vi "Create Icon Layer New.vi"(8 "error in (no error)":errorcluster, 9 "Template data":T5 {"Opacity" scale=0.0..100.0}, 10 "Icon data":T1={"Text Visible?"=FALSE, "Text Opacity"=0, "Templ Visible?"=FALSE, "Templ Opacity"=0, "Relative Path from 1 to 2"=path "", "Image"=bytes[0], "All User Layers"=[], "Body Text"={"Line 1 text"="", "Line 2 text"="", "Line 3 text"="", "Line 4 text"="", "Line 1 color"=0, "Line 2 color"=0, "Line 3 color"=0, "Line 4 color"=0, "Body Text Spec"={"Font"="", "Alignment"=0, "Size"=3}, "Center text vertically"=FALSE, "Capitalize Text"=FALSE}} {"Body Text"."Body Text Spec"."Alignment" items=["left", "center", "right"]}, 11 "Text data":T5 {"Opacity" scale=0.0..100.0}) -> (0 "error out":errorcluster, 3 "Icon out":refnum<class "Icon.lvclass">)   [LabVIEW 2020, in "VI Properties Editor.lvlib"]
doc: "Create an Icon Layer with the given data from the LabVIEW Icon Data."
uses:
  VI Properties Editor.lvlib
  <vilib>/LabVIEW Icon API/lv_icon/Classes/Icon/Icon.lvclass
  <vilib>/LabVIEW Icon API/lv_icon/Classes/Layer/Layer.lvclass
  <vilib>/LabVIEW Icon API/lv_icon/Classes/Icon Framework/Icon Framework.lvclass
  <vilib>/LabVIEW Icon API/lv_icon/Controls/LayerType.ctl
  <vilib>/LabVIEW Icon API/lv_icon/Controls/Graphic.ctl
  <vilib>/LabVIEW Icon API/lv_icon/lv_icon.lvlib
  <vilib>/LabVIEW Icon API/lv_icon/Controls/Pathes.ctl
  <vilib>/LabVIEW Icon API/lv_icon/Controls/Layer.ctl
  <vilib>/LabVIEW Icon API/lv_icon/Controls/Font.ctl
  <vilib>/LabVIEW Icon API/lv_icon/Controls/Alignment.ctl
  <vilib>/LabVIEW Icon API/lv_icon/Controls/BodyText.ctl
  <vilib>/LabVIEW Icon API/lv_icon/Controls/LabVIEW Icon Stored Information.ctl
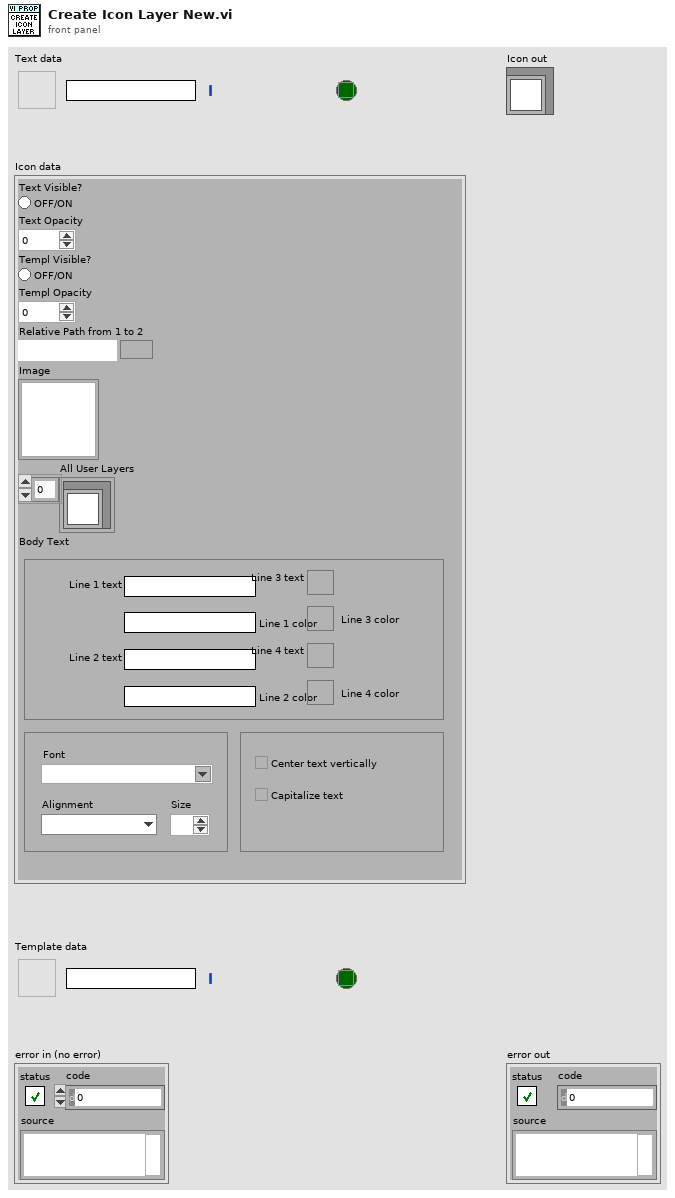
[diagram p1: front panel]
types:
  T1 = typedef "LabVIEW Icon Stored Information.ctl" = cluster{"Text Visible?":bool, "Text Opacity":u8, "Templ Visible?":bool, "Templ Opacity":u8, "Relative Path from 1 to 2":path, "Image":picture, "All User Layers":refnum<class "Layer.lvclass">[], "Body Text":T2}
  T2 = typedef "BodyText.ctl" = cluster{"Line 1 text":string, "Line 2 text":string, "Line 3 text":string, "Line 4 text":string, "Line 1 color":u32, "Line 2 color":u32, "Line 3 color":u32, "Line 4 color":u32, "Body Text Spec":cluster{"Font":T3, "Alignment":T4, "Size":u8}, "Center text vertically":bool, "Capitalize Text":bool}
  T3 = typedef "Font.ctl" = string
  T4 = typedef "Alignment.ctl" = u16
  T5 = typedef "Layer.ctl" = cluster{"LayerIcon":picture, "LayerName":string, "Opacity":u8, "Visibility?":bool}
  T6 = typedef "Pathes.ctl" = enum16{"Root Path", "Icon Templates", "Icon Templates VI", "Icon Templates Lib", "Glyphs"}
  T7 = typedef "Graphic.ctl" = cluster{"Rectangle":cluster{"left":i16, "top":i16, "right":i16, "bottom":i16}, "Path":path, "Image":picture, "Filter":string, "FileName":string}
  T8 = typedef "LayerType.ctl" = enum16{"Graphic", "Text", "Tool", "Graphic Drop"}
  T9 = typedef "imagedata.ctl" = cluster{"image type":i32, "image depth":i32, "image":u8[], "mask":u8[], "colors":u32[], "Rectangle":cluster{"left":i16, "top":i16, "right":i16, "bottom":i16}}
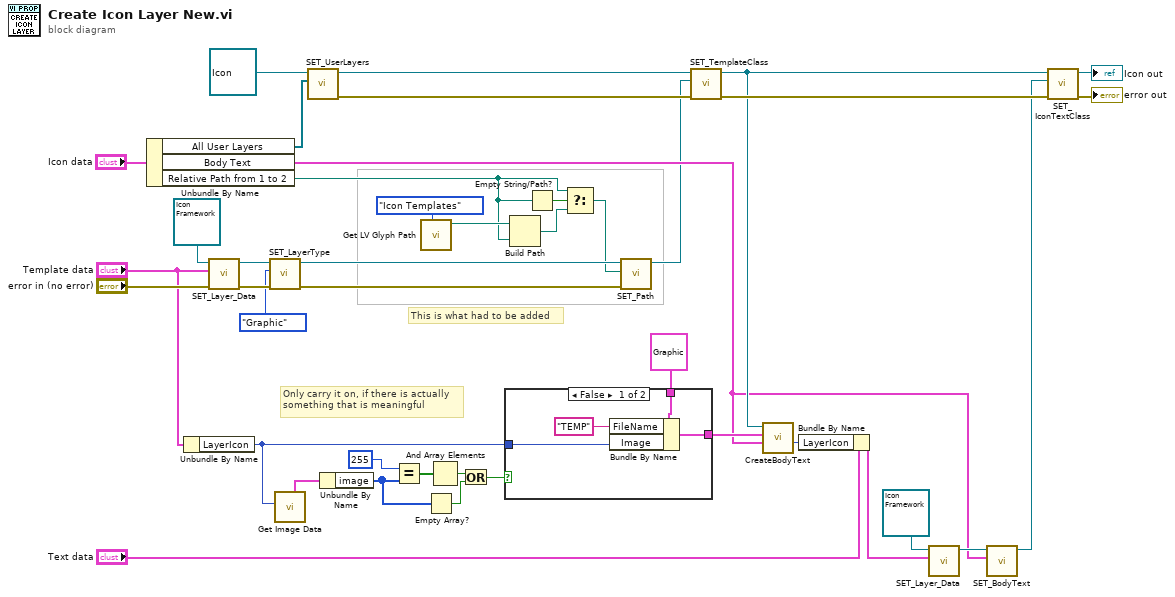
[diagram p0: block diagram]
diagram:
  # "This is what had to be added"
  # "Only carry it on, if there is actually\nsomething that is meaningful"
  n1 = Unbundle By Name("Icon data") -> ("All User Layers"=w32:refnum<class "Layer.lvclass">[], "Body Text"=w22:T2, "Relative Path from 1 to 2"=w3:path)
  n2 = Unbundle By Name("Template data") -> ("LayerIcon"=w12:picture)
  n3 = call-dynamic "SET_Layer_Data.vi"("error in (no error)"="error in (no error)", "Data"="Template data", "Layer.lvclass in"=refnum<class "Icon Framework.lvclass"> refnum ("lv_icon.lvlib:Icon Framework.lvclass")) -> ("error out"=w40:errorcluster, "Layer.lvclass out"=w37:refnum<class "Icon Framework.lvclass">)  [unwired: 1 in, 6 out]
  n4 = call-dynamic "SET_LayerType.vi"("error in (no error)"=w40, "Type"=LayerType."Graphic", "Layer.lvclass in"=w37) -> ("error out"=w9:errorcluster, "Layer.lvclass out"=w8:refnum<class "Icon Framework.lvclass">)  [unwired: 7 out]
  n5 = call <vilib>:"Get Image Data.vi"("Pic In"=w12) -> ("image data out"=w18:T9)  [unwired: 2 in, 8 out]
  n6 = call-dynamic "SET_UserLayers.vi"("Layers"=w32, "Icon.lvclass in"=refnum<class "Icon.lvclass"> refnum ("Icon in")) -> ("error out"=w35:errorcluster, "Icon.lvclass out"=w36:refnum<class "Icon.lvclass">)  [unwired: 8 in]
  n7 = Unbundle By Name(w18) -> ("image"=w14:u8[])
  n8 = Equal?(x=u8 255, y=w14) -> (x = y?=w16:bool[])
  n9 = call <vilib>:"Get LV Glyph Path.vi"("Path"=Pathes."Icon Templates") -> ("Requested Path"=w5:path)  [unwired: 2 in, 8 out]
  n10 = Empty Array?(array=w14) -> (empty?=w13:bool)
  n11 = And Array Elements(Boolean array=w16) -> (logical AND=w15:bool)
  n12 = Or(x=w15, y=w13) -> (x .or. y?=w11:bool)
  n13 = case shown="False" w11 {
    tunnel: [w45 w46] -> w26
    tunnel: w12 -> [w44 _]
    tunnel: T7 {"Rectangle"={"left"=0, "top"=0, "right"=0, "bottom"=0}, "Path"=path "", "Image"=bytes[0], "Filter"="", "FileName"=""} ("Path and Icon Template") -> [w43 w46]
    frame False {
      n14 = Bundle By Name(cluster=w43, "FileName"="TEMP", "Image"=w44) -> (w45:T7)
    }
    frame True {
    }
  }
  n15 = Build Path(base path=w5, name or relative path=w3) -> (appended path=w2:path)
  n16 = Empty String/Path?(string/path=w3) -> (empty?=w4:bool)
  n17 = Select(t=w3, s=w4, f=w2) -> (s? t:f=w1:path)
  n18 = call <vilib>:"SET_Path.vi"("error in (no error)"=w9, "Path"=w1, "Icon Framework.lvclass in"=w8) -> ("Icon Framework.lvclass out"=w7:refnum<class "Icon Framework.lvclass">)  [unwired: 7 in, 1 out]
  n19 = call-dynamic "SET_TemplateClass.vi"("error in (no error)"=w35, "Icon Framework.lvclass"=w7, "Icon.lvclass in"=w36) -> ("error out"=w29:errorcluster, "Icon.lvclass out"=w28:refnum<class "Icon.lvclass">)  [unwired: 7 out]
  n20 = call <vilib>:"CreateBodyText.vi"("Body Text"=w22, "Path and Icon Template"=w26, "Icon.lvclass in"=w28) -> ("Body Text"=w23:picture)  [unwired: 8 in]
  n21 = Bundle By Name(cluster="Text data", "LayerIcon"=w23) -> (w24:T5)
  n22 = call-dynamic "SET_Layer_Data.vi"("Data"=w24, "Layer.lvclass in"=refnum<class "Icon Framework.lvclass"> refnum ("lv_icon.lvlib:Icon Framework.lvclass")) -> ("Layer.lvclass out"=w31:refnum<class "Icon Framework.lvclass">)  [unwired: 8 in, 1 out]
  n23 = call-dynamic "SET_BodyText.vi"("Body Text"=w22, "Icon Framework.lvclass in"=w31) -> ("Icon Framework.lvclass out"=w21:refnum<class "Icon Framework.lvclass">)  [unwired: 8 in, 1 out]
  n24 = call-dynamic "SET_IconTextClass.vi"("error in (no error)"=w29, "Icon Framework.lvclass"=w21, "Icon.lvclass in"=w28) -> ("error out"=→"error out":errorcluster, "Icon.lvclass out"=→"Icon out":refnum<class "Icon.lvclass">)  [unwired: 7 out]
